vi "PSVCH_Check.vi"(8 "Error In (no error)":errorcluster, 10 "VarList":cluster{"Tag":string[], "Name":string[]}, 11 "Formula":string) -> (0 "Error Out":errorcluster, 1 "Formula Node out":T1, 2 "source":string, 3 "code":i32, 5 "VarList":T5)   [LabVIEW 2016]
uses:
  Private/Ctrls/PSVCH_VarList.ctl
  ToolKit/Formula/Ctrls/PSFormula_FOR_Formula Node.ctl
  ToolKit/Formula/Ctrls/PSFormula_FOR_Formula Step.ctl
  ToolKit/Formula/Ctrls/PSFormula_FOR_Formula Para.ctl
  ToolKit/Formula/Ctrls/PSFormula_FOR_Formula MidVar Data.ctl
panel:
  # "Data In"
  # "Data Out"
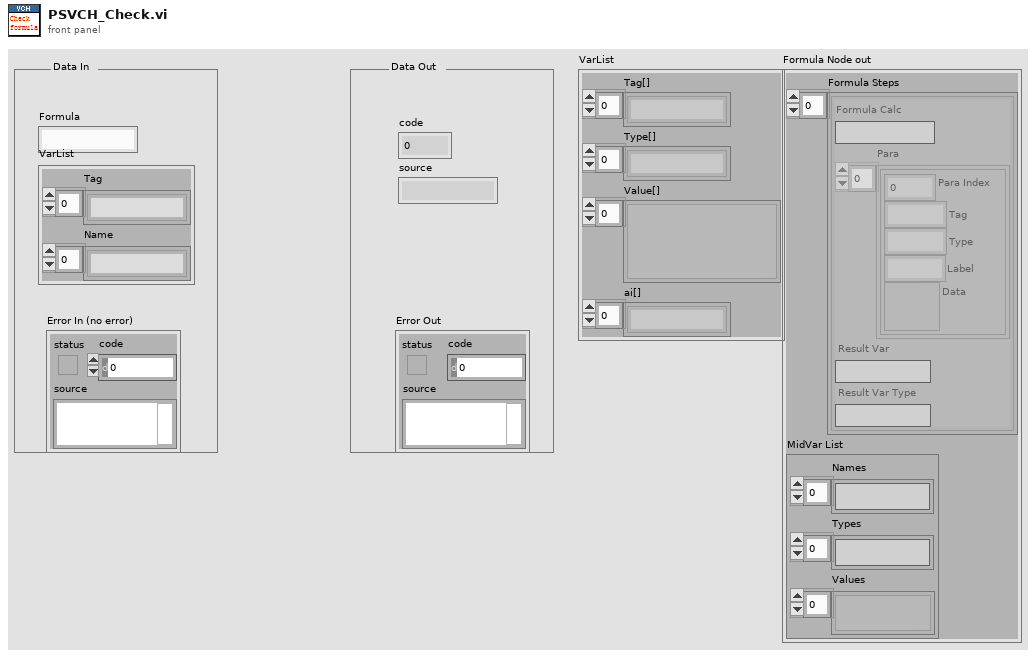
[diagram p1: front panel]
types:
  T1 = typedef "PSFormula_FOR_Formula Node.ctl" = cluster{"Formula Steps":T2[], "MidVar List":T4}
  T2 = typedef "PSFormula_FOR_Formula Step.ctl" = cluster{"Formula Calc":string, "Para":T3[], "Result Var":string, "Result Var Type":string}
  T3 = typedef "PSFormula_FOR_Formula Para.ctl" = cluster{"Para Index":i32, "Tag":string, "Type":string, "Label":string, "Data":variant}
  T4 = typedef "PSFormula_FOR_Formula MidVar Data.ctl" = cluster{"Names":string[], "Types":string[], "Values":variant[]}
  T5 = typedef "PSVCH_VarList.ctl" = cluster{"Tag[]":string[], "Type[]":string[], "Value[]":variant[], "ai[]":string[]}
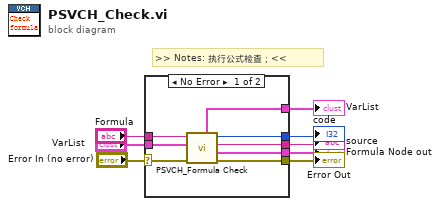
[diagram p0: block diagram]
diagram:
  # ">> Notes: 执行公式检查；<<"
  n1 = case shown="No Error" "Error In (no error)" {
    selector: "Error In (no error)" -> [w16 w17]
    tunnel: [w14 w17] -> w7
    tunnel: "Formula" -> [w15 _]
    tunnel: [w13 _] -> w5
    tunnel: [w12 _] -> w4
    tunnel: "VarList" -> [w11 _]
    tunnel: [w10 _] -> w1
    tunnel: [w9 _] -> w2
    frame No Error {
      n2 = call "PSVCH_Formula Check.vi"("Error In"=w16, "VarList"=w11, "Formula"=w15) -> ("Error Out"=w14:errorcluster, "Formula Node out"=w10:T1, "source"=w12:string, "code"=w13:i32, "VarList"=w9:T5)  [unwired: 4 in]
    }
    frame Error {
    }
  }
  "Error Out" <- w7
  "code" <- w5
  "source" <- w4
  "VarList" <- w2
  "Formula Node out" <- w1
